vi "motorPID.vi"(2 "PID gains":T1={"proportional gain (Kc)"=0.3, "integral time (Ti, min)"=0.0, "derivative time (Td, min)"=0.0001}, 3 "output range":cluster{"output high":dbl, "output low":dbl}={"output high"=100.0, "output low"=-100.0}, 7 "目標":dbl[](array[numeric]), 9 "dt (s)":dbl=0.010000000000000002 format="%#_13g", 11 "error in (no error)":errorcluster, 12 "reinitialize? (F)":bool, 13 "EncRst":bool) -> (8 "power":dbl[](array[numeric]), 10 "Enc":dbl[](array[numeric]), 14 "差值":dbl[](array[numeric]), 15 "error out":errorcluster)   [LabVIEW 2019]
uses:
  <vilib>/addons/control/pid/pid.llb/PID (DBL).vi
  <vilib>/addons/control/pid/NI_PID_pid.lvlib
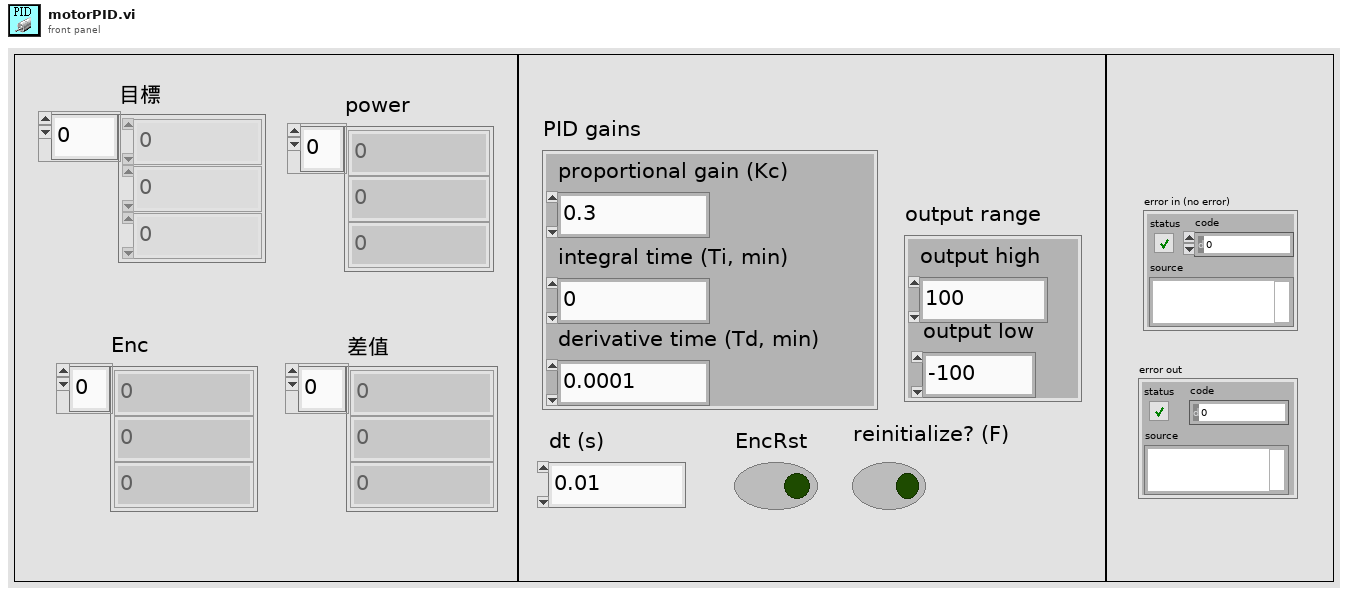
[diagram p1: front panel]
types:
  T1 = cluster{"proportional gain (Kc)":dbl, "integral time (Ti, min)":dbl, "derivative time (Td, min)":dbl}
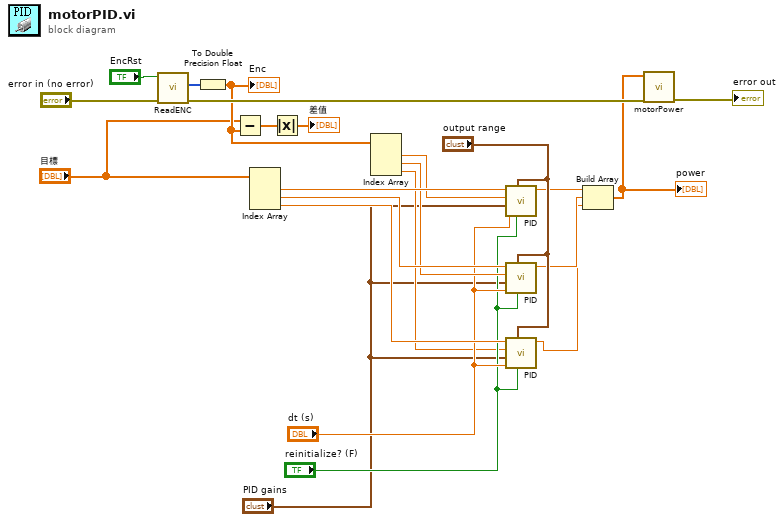
[diagram p0: block diagram]
diagram:
  n1 = call "ReadENC.vi"("error in (no error)"="error in (no error)", "Reset"="EncRst") -> ("error out"=w14:errorcluster, "ENC"=w11:i32[])  [unwired: 8 in]
  n2 = To Double Precision Float(number=w11) -> (double precision float=w5:dbl[])
  "Enc" <- w5
  n3 = Subtract(x="目標", y=w5) -> (x-y=w18:dbl[])
  n4 = Index Array(array="目標") -> (element #1=w23:dbl, element #2=w22:dbl, element #3=w21:dbl)  [unwired: 3 in]
  n5 = Absolute Value(x=w18) -> (abs(x)=→"差值":dbl[])
  n6 = Index Array(array=w5) -> (element #1=w20:dbl, element #2=w19:dbl, element #3=w7:dbl)  [unwired: 3 in]
  n7 = call-poly <vilib>:"PID.vi"("reinitialize? (F)"="reinitialize? (F)", "output range"="output range", "dt (s)"="dt (s)", "PID gains"="PID gains", "process variable"=w20, "setpoint"=w23) -> ("output"=w2:dbl)  [unwired: 4 in, 1 out]
  n8 = call-poly <vilib>:"PID.vi"("reinitialize? (F)"="reinitialize? (F)", "output range"="output range", "dt (s)"="dt (s)", "PID gains"="PID gains", "process variable"=w19, "setpoint"=w22) -> ("output"=w3:dbl)  [unwired: 4 in, 1 out]
  n9 = call-poly <vilib>:"PID.vi"("reinitialize? (F)"="reinitialize? (F)", "output range"="output range", "dt (s)"="dt (s)", "PID gains"="PID gains", "process variable"=w7, "setpoint"=w21) -> ("output"=w1:dbl)  [unwired: 4 in, 1 out]
  n10 = Build Array(w2, w3, w1) -> (w12:dbl[])
  "power" <- w12
  n11 = call "motorPower.vi"("error in (no error)"=w14, "DC_Pwr"=w12) -> ("error out"=→"error out":errorcluster)  [unwired: 9 in]
